vi "Get Next.vi"(0 "Executioner in":refnum<class "Executioner.lvclass">, 1 "Linked List Ref":refnum<data-value>, 5 "Active Unique ID":string, 9 "Active Element Index":i32, 11 "error in (no error)":errorcluster) -> (3 "Linked List Ref out":refnum<data-value>, 4 "Executioner out":refnum<class "Executioner.lvclass">, 6 "Active Unique ID out":string, 8 "Test Executive Ref out":refnum<data-value>, 10 "Active Element Index out":i32, 12 "Found":bool, 13 "Complete":bool, 14 "Stop":bool, 15 "error out":errorcluster)   [LabVIEW 2017, in "Test Executive.lvlib" / "Executioner.lvclass"]
uses:
  <vilib>/gpm_packages/@cs/test-executive/Source/Test Executive/Executioner/Executioner.lvclass
  <vilib>/gpm_packages/@cs/linked-list/Source/Linked List/ILinkedList/ILinked List.lvclass
  <vilib>/gpm_packages/@cs/test-executive/Source/Test Executive/ITestExecutive/ITest Executive.lvclass
  <vilib>/gpm_packages/@cs/linked-list/Source/Linked List/Linked List Ref/Linked List Ref.lvclass
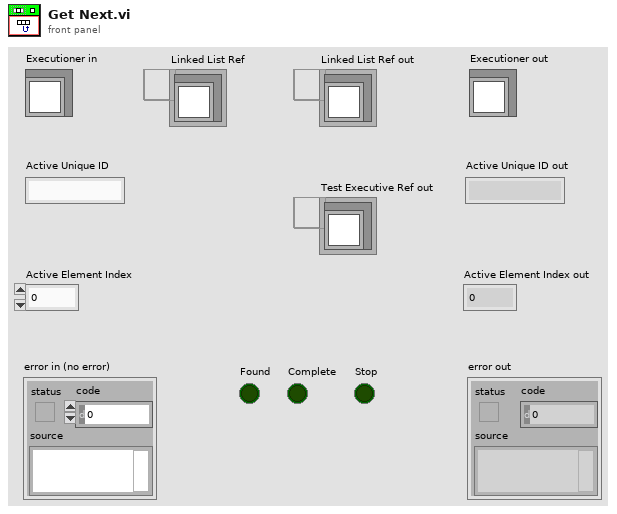
[diagram p1: front panel]
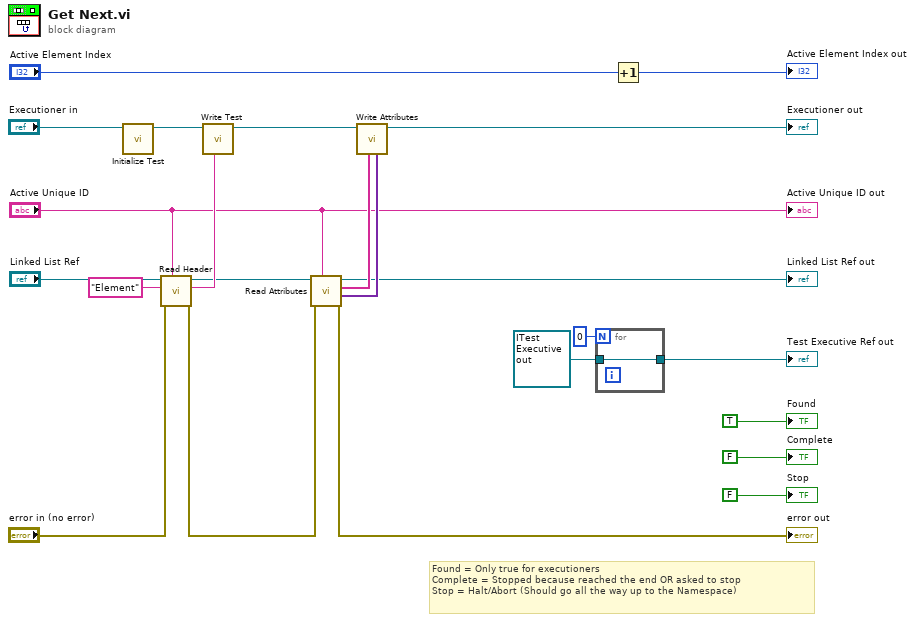
[diagram p0: block diagram]
diagram:
  # "Found = Only true for executioners\nComplete = Stopped because reached the end OR asked to stop\nStop = Halt/Abort (Should go all the way up to the Namespace)"
  n1 = call <vilib>:"Initialize Test.vi"("Executioner in"="Executioner in") -> ("Executioner out"=w4:refnum<class "Executioner.lvclass">)  [unwired: 10 in]
  n2 = call <vilib>:"Read Header.vi"("Linked List ID"="Active Unique ID", "error in (no error)"="error in (no error)", "Header Name"="Element", "Linked List Ref"="Linked List Ref") -> ("error out"=w16:errorcluster, "Header Value"=w18:string, "Linked List Ref out"=w17:refnum<data-value>)  [unwired: 4 in, 1 out]
  n3 = call <vilib>:"Write Test.vi"("Test"=w18, "Executioner in"=w4) -> ("Executioner out"=w23:refnum<class "Executioner.lvclass">)  [unwired: 9 in]
  n4 = call <vilib>:"Read Attributes.vi"("Linked List ID"="Active Unique ID", "error in (no error)"=w16, "Linked List Ref"=w17) -> ("error out"=→"error out":errorcluster, "Attributes"=w13:variant[], "Attribute Names out"=w14:string[], "Linked List Ref out"=→"Linked List Ref out":refnum<data-value>)  [unwired: 3 in, 2 out]
  n5 = call <vilib>:"Write Attributes.vi"("Attributes"=w13, "Attribute Names"=w14, "Executioner in"=w23) -> ("Executioner out"=→"Executioner out":refnum<class "Executioner.lvclass">)  [unwired: 8 in]
  n6 = for {
    N: 0 -> [_]
    tunnel: refnum<data-value> refnum ("Test Executive Ref out") -> [w24]
    tunnel: [w24] -> w1
  }
  "Test Executive Ref out" <- w1
  n7 = Increment(x="Active Element Index") -> (x+1=→"Active Element Index out":i32)
  "Active Unique ID out" <- "Active Unique ID"
  "Found" <- TRUE ("Found")
  "Complete" <- FALSE ("Complete")
  "Stop" <- FALSE ("Stop")
